vi "未命名 2 (子VI).vi"() -> (0 "错误输出":errorcluster, 3 "引用句柄输出":refnum<k20> caption="FPGA VI引用输出")   [LabVIEW 2017]
uses:
  <vilib>/FPGAPlugInAG/myRIO-1900/niLvFpga_Open_myRIO-1900.vi
  <vilib>/rvi/interface/common/dynamic/niFpgaDynamicAddResources.vi
  <vilib>/rvi/interface/nirviOpenFPGA/nirviOpenFPGA.xnode
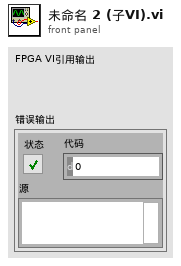
[diagram p1: front panel]
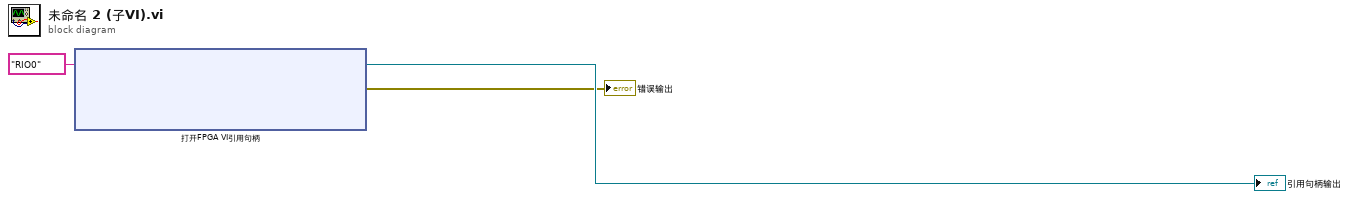
[diagram p0: block diagram]
diagram:
  n1 = xnode "打开FPGA VI引用句柄"("资源名称"=tag "RIO0") -> ("FPGA VI引用输出"=→"引用句柄输出":refnum<k20>, "错误输出"=→"错误输出":errorcluster)  [unwired: 1 in]
